vi "Test vi.vi"() -> ()   [LabVIEW 2016]
uses:
  Libraries/User Interface/AI Channel Setting.ctl
  <vilib>/DAQmx/read.llb/DAQmx Read (Analog 1D Wfm NChan NSamp).vi
  <vilib>/DAQmx/miscellaneous.llb/DAQmx Fill In Error Info.vi
  Libraries/DAQ Hardware/DAQ Hardware.lvlib
  <resource>/objmgr/daqmx.rc
panel:
  out "Waveform":waveform(dbl)
  in  "Boolean":bool
  out "dt":dbl
  out "x-y":u32
  in  "error in (no error)":errorcluster
  out "error out":errorcluster
  out "data":waveform(dbl)[](array[waveform])
  in  "AI Setting":T1={"Physical Channel"=["6363/ai0", "6363/ai1", "6363/ai2"], "Name to assign"=["Analog input1", "Analog input2", "Analog input3"], "input terminal configuration"=enum."RSE", "minimum value"=0.0, "maximum value"=10.0, "units"=enum."Volts", "custom scale name"="", "sample mode"=enum."Finite Samples", "rate"=5000.0, "samples per channel"=1000} {"rate" format="%#_13g"; "maximum value" format="%#_13g"; "minimum value" format="%#_13g"}
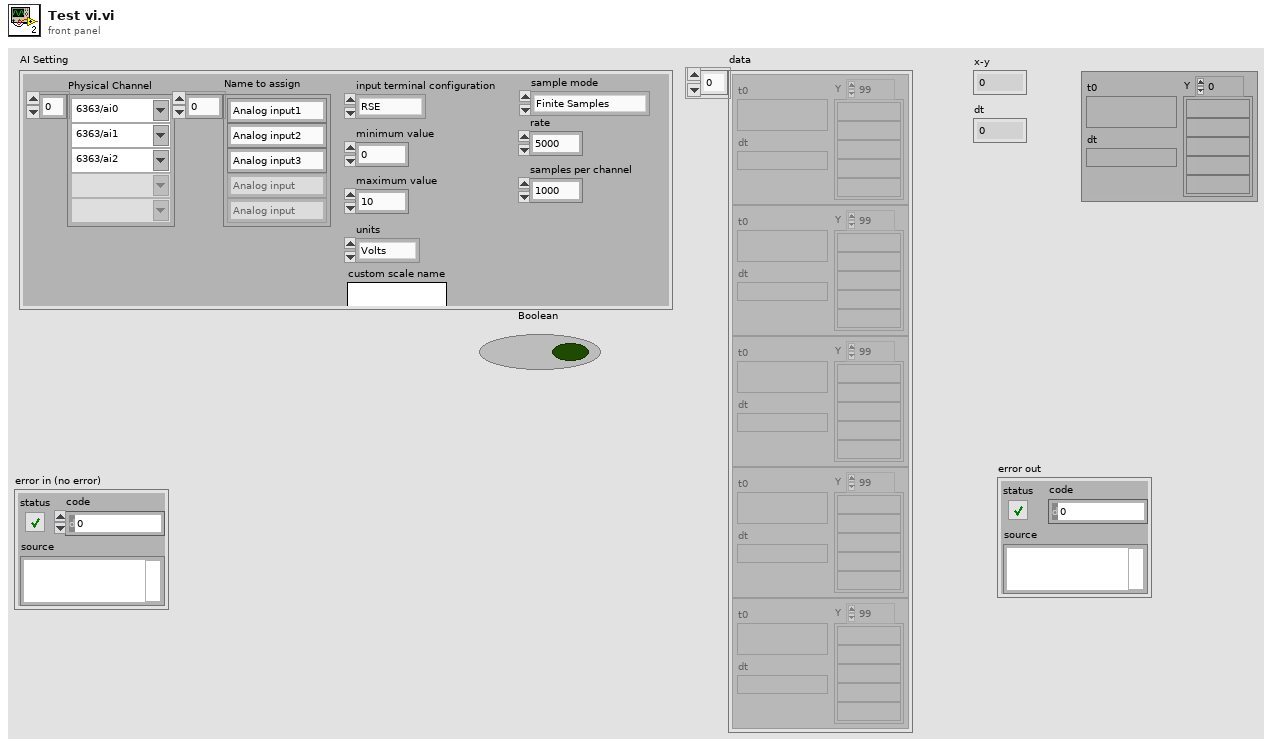
[diagram p1: front panel]
types:
  T1 = typedef "DAQ Hardware.lvlib/AI Channel Setting.ctl" = cluster{"Physical Channel":string[], "Name to assign":string[], "input terminal configuration":enum16{"RSE", "NRSE", "Differential"}, "minimum value":dbl, "maximum value":dbl, "units":enum16{"Volts"}, "custom scale name":string, "sample mode":enum16{"Finite Samples", "Continuous Samples", "Hardware Timed Single Point"}, "rate":dbl, "samples per channel":i32}
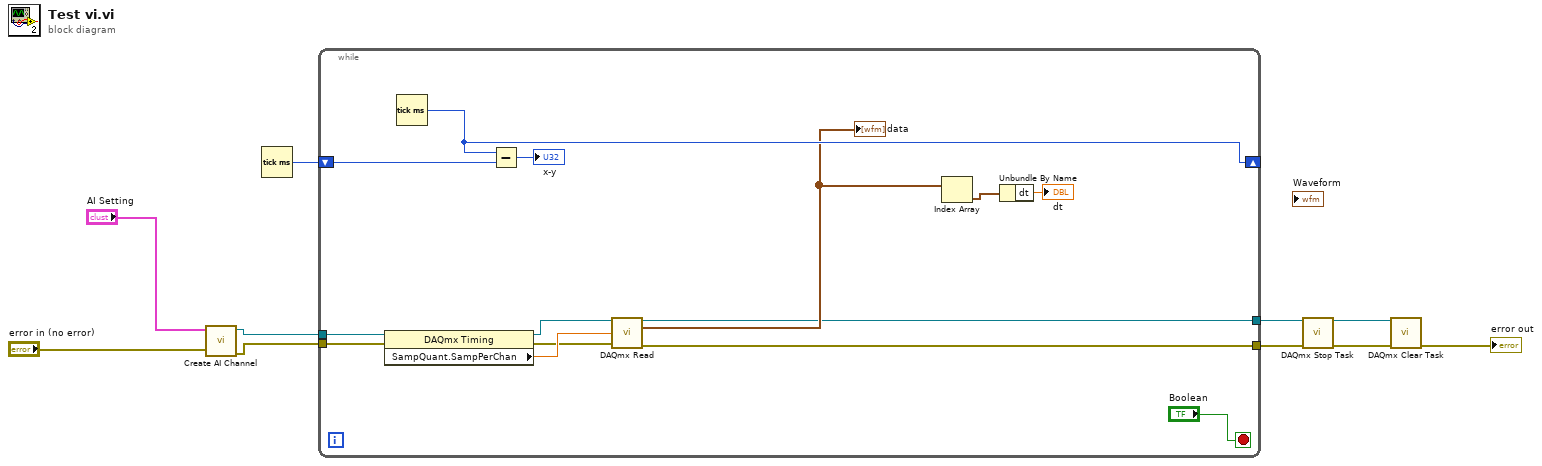
[diagram p0: block diagram]
diagram:
  n1 = call "Create AI Channel.vi"("error in (no error)"="error in (no error)", "AI Setting"="AI Setting") -> ("error out"=w9:errorcluster, "task out"=w8:refnum<k21>)  [unwired: 8 in]
  n2 = Tick Count (ms)() -> (millisecond timer value=w6:u32)
  n3 = while {
    tunnel: w9 -> [w21]
    tunnel: w8 -> [w20]
    tunnel: [w16] -> w5
    shift-right: [w15] -> _
    shift-left: w6 -> [w18]
    tunnel: [w11] -> w2
    stop <- "Boolean" stop-if-true
    n4 = property class="DAQmx Timing"(reference=w20, error in=w21) -> (reference out=w23:refnum<k21>, error out=w22:errorcluster, "SampQuant.SampPerChan"=w24:dbl)
    n5 = Tick Count (ms)() -> (millisecond timer value=w15:u32)
    n6 = Subtract(x=w15, y=w18) -> (x-y=→"x-y":u32)
    n7 = call-poly <vilib>:"DAQmx Read.vi"("task/channels in"=w23, "number of samples per channel"=w24, "error in"=w22) -> ("task out"=w11:refnum<k21>, "data"=w14:waveform(dbl)[], "error out"=w16:errorcluster)  [unwired: 10 in]
    "data" <- w14
    n8 = Index Array(array=w14) -> (element=w13:waveform(dbl))  [unwired: 1 in]
    n9 = Unbundle By Name(w13) -> ("dt"=→"dt":dbl)
  }
  n10 = call <vilib>:"DAQmx Stop Task.vi"("task/channels in"=w2, "error in"=w5) -> ("task out"=w1:refnum<k21>, "error out"=w4:errorcluster)  [unwired: 12 in]
  n11 = call <vilib>:"DAQmx Clear Task.vi"("task in"=w1, "error in"=w4) -> ("error out"=→"error out":errorcluster)  [unwired: 13 in]
